vi "PrintError.vi"(8 "error in (no error)":errorcluster) -> (0 "error out":errorcluster)   [LabVIEW 2016, in "Log4Lv.lvlib"]
doc: "Use this template to build a VI to use as a subVI."
uses:
  Log4Lv.lvlib
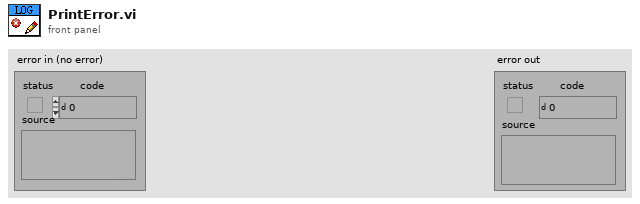
[diagram p1: front panel]
types:
  T1 = enum16{"Disable", "Error", "Warn", "Info", "Debug"}
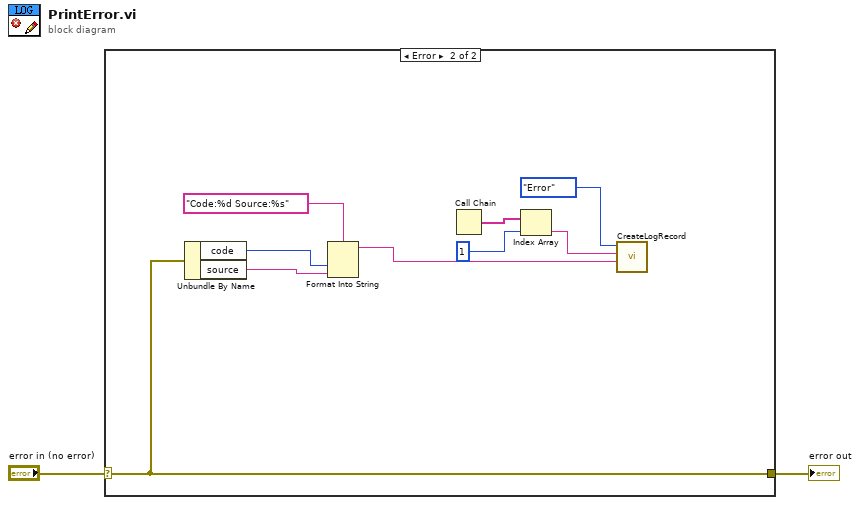
[diagram p0: block diagram]
diagram:
  n1 = case shown="Error" "error in (no error)" {
    selector: "error in (no error)" -> [w3 w12]
    tunnel: [w3 w12] -> w1
    frame No Error {
    }
    frame Error {
      n2 = Unbundle By Name(w12) -> ("code"=w11:i32, "source"=w9:string)
      n3 = Format Into String(format string="Code:%d Source:%s", w11, w9) -> (resulting string=w4:string)  [unwired: 2 in, 1 out]
      n4 = Call Chain() -> (call chain=w7:string[])
      n5 = Index Array(array=w7, index=1) -> (element=w6:string)
      n6 = call "CreateLogRecord.vi"("Message"=w4, "Source"=w6, "Level"=T1."Error") -> ()  [unwired: 8 in, 1 out]
    }
  }
  "error out" <- w1
